vi "SVXMPL_Two Axis Acceleometer (simulated).vi"(6 "sampling info":cluster{"Fs":dbl, "#s":dbl}={"Fs"=51200.0, "#s"=8192.0} {"#s" format="%.2p"; "Fs" format="%.2p"}, 7 "noise amplitude":dbl=0.01 format="%.2f", 8 "error in (no error)":errorcluster, 10 "Y Axis Accelerometer":T1={"fundamental"=25.0, "Amplitude"=1.0, "phase"=90.0, "harmonics"=enum."odd only", "# of harmonics"=8} {"phase" format="%.2f"; "Amplitude" format="%.2f"; "fundamental" format="%.2f"}, 11 "X Axis Accelerometer":T1={"fundamental"=25.0, "Amplitude"=1.0, "phase"=0.0, "harmonics"=enum."odd only", "# of harmonics"=4} {"phase" format="%.2f"; "Amplitude" format="%.2f"; "fundamental" format="%.2f"}) -> (0 "error out":errorcluster, 3 "signal out":waveform(dbl)[](array[waveform])=[{"t0"=timestamp(0 s since 1904-01-01), "dt"=1.953125e-05, "Y"=array[8192 elements]}, {"t0"=timestamp(0 s since 1904-01-01), "dt"=1.953125e-05, "Y"=array[8192 elements]}])   [LabVIEW 2017]
panel:
  out "Waveform Graph 2":waveform(dbl)[](graph)=[{"t0"=timestamp(0 s since 1904-01-01), "dt"=1.953125e-05, "Y"=array[8192 elements]}, {"t0"=timestamp(0 s since 1904-01-01), "dt"=1.953125e-05, "Y"=array[8192 elements]}]
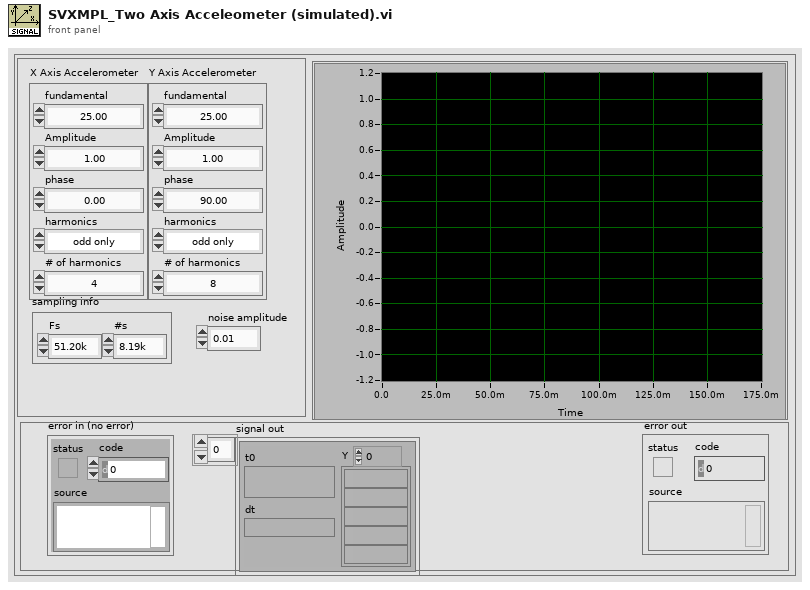
[diagram p1: front panel]
types:
  T1 = cluster{"fundamental":dbl, "Amplitude":dbl, "phase":dbl, "harmonics":enum16{"All", "odd only", "even only", "Custom frequencies"}, "# of harmonics":i32}
  T2 = enum16{"All", "odd only", "even only", "Custom frequencies"}
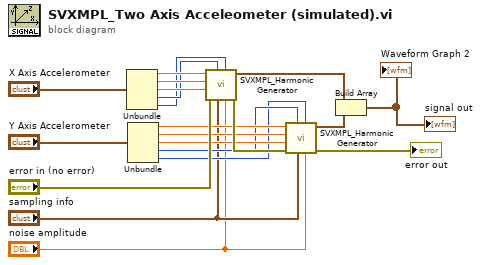
[diagram p0: block diagram]
diagram:
  n1 = Unbundle("X Axis Accelerometer") -> ("fundamental"=w15:dbl, "Amplitude"=w14:dbl, "phase"=w13:dbl, "harmonics"=w12:T2, "# of harmonics"=w11:i32)
  n2 = Unbundle("Y Axis Accelerometer") -> ("fundamental"=w10:dbl, "Amplitude"=w9:dbl, "phase"=w8:dbl, "harmonics"=w7:T2, "# of harmonics"=w6:i32)
  n3 = call <vilib>:"SVXMPL_Harmonic Generator.vi"("noise amplitude"="noise amplitude", "# of harmonics"=w11, "sampling info"="sampling info", "harmonics"=w12, "error in (no error)"="error in (no error)", "phase"=w13, "Amplitude"=w14, "fundamental"=w15) -> ("error out"=w16:errorcluster, "Waveform"=w2:waveform(dbl))  [unwired: 2 in]
  n4 = call <vilib>:"SVXMPL_Harmonic Generator.vi"("noise amplitude"="noise amplitude", "# of harmonics"=w6, "sampling info"="sampling info", "harmonics"=w7, "error in (no error)"=w16, "phase"=w8, "Amplitude"=w9, "fundamental"=w10) -> ("error out"=→"error out":errorcluster, "Waveform"=w17:waveform(dbl))  [unwired: 2 in]
  n5 = Build Array(w2, w17) -> (→"signal out" →"Waveform Graph 2":waveform(dbl)[])
